vi "_Strip apostrophe - Element.vi"(11 "string":string) -> (3 "s? t:f":string)   [LabVIEW 2017]
uses:
  <userlib>/_OpenG.lib/string/string.llb/Trim Whitespace (String)__ogtk.vi
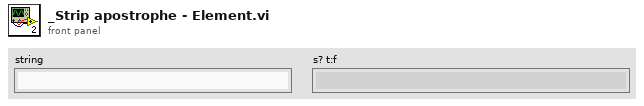
[diagram p1: front panel]
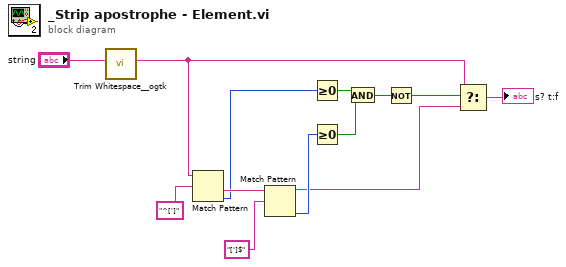
[diagram p0: block diagram]
diagram:
  n1 = call-poly <userlib>:"Trim Whitespace__ogtk.vi"("String in"="string") -> ("String out"=w1:string)  [unwired: 6 in]
  n2 = Match Pattern(string=w1, regular expression="^[']") -> (after substring=w12:string, offset past match=w10:i32)  [unwired: 1 in, 2 out]
  n3 = Match Pattern(string=w12, regular expression="[']$") -> (before substring=w4:string, offset past match=w9:i32)  [unwired: 1 in, 2 out]
  n4 = Greater Or Equal To 0?(x=w10) -> (x >= 0?=w8:bool)
  n5 = Greater Or Equal To 0?(x=w9) -> (x >= 0?=w7:bool)
  n6 = And(x=w8, y=w7) -> (x .and. y?=w6:bool)
  n7 = Not(x=w6) -> (.not. x?=w3:bool)
  n8 = Select(t=w1, s=w3, f=w4) -> (s? t:f=→"s? t:f":string)
